vi "Net Time Changed.vi"(4 "User Parameter":T1, 5 "Event Data":cluster{"sender":refnum<k24>, "e":refnum<k24>}, 6 "Control Ref":refnum<k24>, 7 "Event Common Data":T2) -> ()   [LabVIEW 2021]
uses:
  System.Windows.Forms
  tdefs/td.Message.ctl
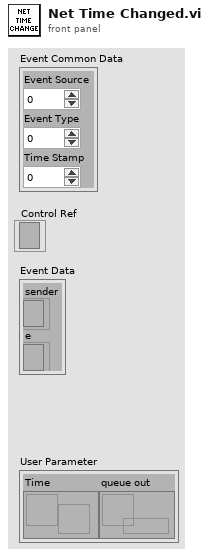
[diagram p1: front panel]
types:
  T1 = cluster{"Time":refnum<user-event>, "queue out":refnum<queue>}
  T2 = cluster{"Event Source":i32, "Event Type":u32, "Time Stamp":u32}
  T3 = typedef "td.Message.ctl" = cluster{"Command":string, "Data":variant}
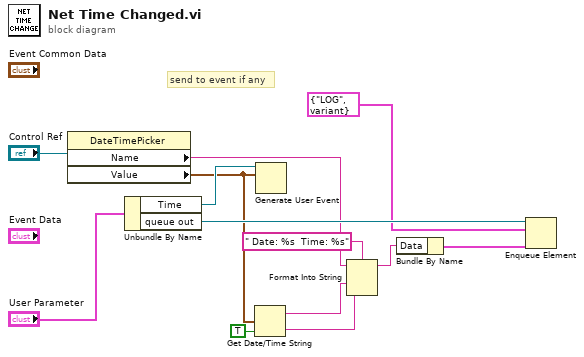
[diagram p0: block diagram]
diagram:
  # "send to event if any"
  n1 = property class="DateTimePicker"(reference="Control Ref") -> ("Name"=w8:string, "Value"=w6:timestamp)  [unwired: 1 in, 2 out]
  n2 = Unbundle By Name("User Parameter") -> ("Time"=w11:refnum<user-event>, "queue out"=w10:refnum<queue>)
  n3 = Get Date/Time String(seconds (now)=w6, want seconds? (F)=TRUE) -> (date string=w4:string, time string=w3:string)  [unwired: 1 in]
  n4 = Generate User Event(user event=w11, event data cluster=w6) -> ()  [unwired: 2 in, 2 out]
  n5 = Format Into String(format string=" Date: %s  Time: %s", initial string=w8, w4, w3) -> (resulting string=w1:string)  [unwired: 1 in, 1 out]
  n6 = Bundle By Name(cluster=T3 {"Command"="LOG", "Data"=variant} ("element"), "Data"=w1) -> (w2:T3)
  n7 = Enqueue Element(queue=w10, element=w2) -> ()  [unwired: 2 in, 3 out]
